vi "Increment Semaphore Ref Name.vi"(8 "error in":errorcluster) -> (0 "error out":errorcluster, 2 "appendStr":string)   [LabVIEW 2015, in "Serial IO.lvclass"]
doc: "Provide a unique name for the semaphore so that we don't have issues with using the same semaphore with different devices. This VI will generate a '_#' which will indicate the number of the semaphore. This would be useful in the case where there might be multiple Alicat Comm banks or TE Coolers talking to the same controller. This VI is global and"
uses:
  Serial IO.lvclass
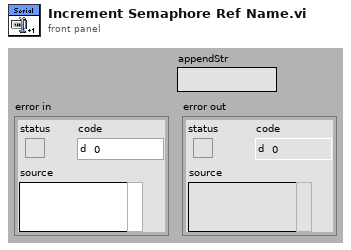
[diagram p1: front panel]
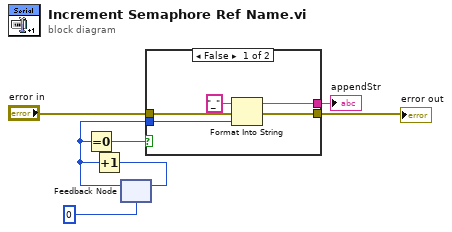
[diagram p0: block diagram]
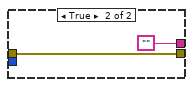
[diagram p2: hidden frame]
diagram:
  n1 = feedback #1(0) -> (w3:i32)
  n2 = Equal To 0?(x=w3) -> (x = 0?=w7:bool)
  n3 = Increment(x=w3) -> (x+1=w6:i32)
  n4 = feedback-in #1(w6) -> ()
  n5 = case shown="False" w7 {
    tunnel: w3 -> [w12 _]
    tunnel: [w10 ""] -> w4
    tunnel: "error in" -> [w9 w13]
    tunnel: [w8 w13] -> w1
    frame False {
      n6 = Format Into String(initial string="_", error in=w9, w12) -> (resulting string=w10:string, error out=w8:errorcluster)  [unwired: 1 in]
    }
    frame True {
    }
  }
  "error out" <- w1
  "appendStr" <- w4
